vi "fish out prompt.vi"(2 "error in":errorcluster, 3 "input string":string) -> (0 "error out":errorcluster, 1 "prompt before $ sign":string)   [LabVIEW 2016, in "labssh_thijs.lvlib"]
uses:
  <vilib>/regexp/Match Regular Expression.xnode
  labssh_thijs.lvlib
panel:
  out "whole match 2":string
  out "prompt and space":string
  out "after match":string
  out "whole match":string
  out "before match":string
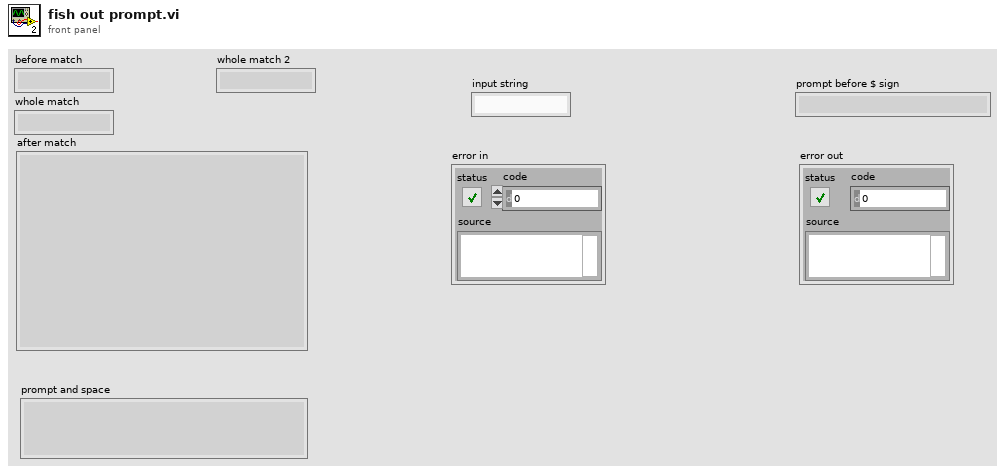
[diagram p1: front panel]
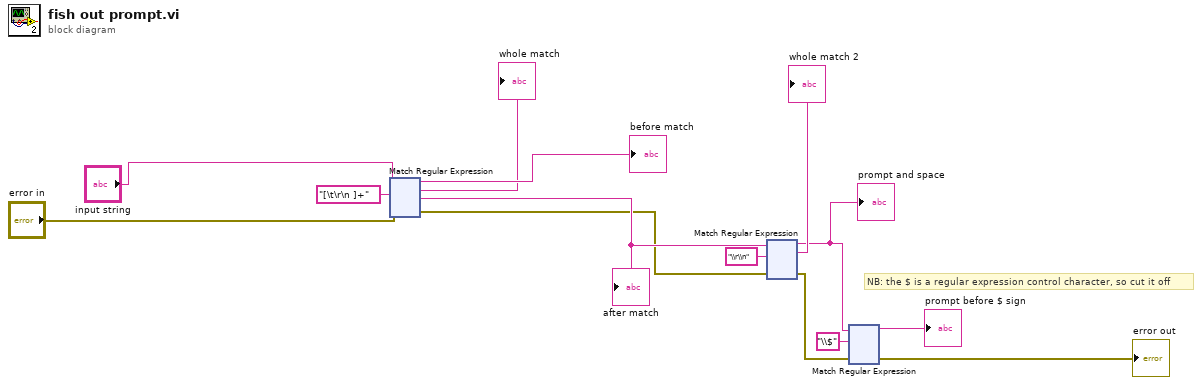
[diagram p0: block diagram]
diagram:
  # "NB: the $ is a regular expression control character, so cut it off"
  n1 = xnode "Match Regular Expression"("input string"="input string", "regular expression"="[\t\r\n ]+", "error in"="error in") -> ("before match"=→"before match":string, "whole match"=→"whole match":string, "after match"=w11:string, "error out"=w4:errorcluster)  [unwired: 3 in, 1 out]
  "after match" <- w11
  n2 = xnode "Match Regular Expression"("input string"=w11, "regular expression"="\\r\\n", "error in"=w4) -> ("before match"=w8:string, "whole match"=→"whole match 2":string, "error out"=w3:errorcluster)  [unwired: 3 in, 2 out]
  "prompt and space" <- w8
  n3 = xnode "Match Regular Expression"("input string"=w8, "regular expression"="\\$", "error in"=w3) -> ("before match"=→"prompt before $ sign":string, "error out"=→"error out":errorcluster)  [unwired: 3 in, 3 out]
